vi "log analysis_gps.vi"() -> ()   [LabVIEW 2018] (continued)
471d,15824;INS_ALIGNMENT_COMPLETE,INS_RTKFIXED,37.37103636428,126.72354662832,8.3755,22.3000,0.1350,-0.2615,-0.0053,-0.069883534,-0.948015743,292.302597203,0.4446,0.2951,0.5590,0.1140,0.0925,0.0776,0.0978,0.1028,4.9465,0f000001,0*59130eb8\n\t", "INSPVAXA,USB3,0,51.0,FINESTEERING,2107,283021.700,02000000,471d,15824;INS_ALIGNMENT_COMPLETE,INS_RTKFIXED,37.37105488806,126.72349758761,8.3107,22.3000,0.1124,-0.2877,-0.0191,-0.603845157,-1.428014368,288.935954178,0.4473,0.2957,0.5615,0.1144,0.0929,0.0777,0.0976,0.1028,4.9397,0f000001,0*95301355\n\t", "INSPVAXA,USB3,0,49.5,FINESTEERING,2107,283026.200,02000000,471d,15824;INS_ALIGNMENT_COMPLETE,INS_RTKFIXED,37.37105960737,126.72348434447,8.2980,22.3000,0.1329,-0.2636,-0.0189,0.063004840,-0.340709655,286.479818282,0.4478,0.2967,0.5618,0.1144,0.0930,0.0777,0.0976,0.1028,4.9376,0f000001,0*1276055f\n\t", "INSPVAXA,USB3,0,49.5,FINESTEERING,2107,283026.700,02000000,471d,15824;INS_ALIGNMENT_COMPLETE,INS_RTKFIXED,37.37106011573,126.72348287105,8.2978,22.3000,0.1361,-0.2641,-0.0054,0.117267102,-0.429574615,286.158968157,0.4478,0.2967,0.5618,0.1144,0.0930,0.0777,0.0976,0.1028,4.9376,0f000001,0*5e7b6e4c\n\t", "INSPVAXA,USB3,0,51.0,FINESTEERING,2107,283028.700,02000000,471d,15824;INS_ALIGNMENT_COMPLETE,INS_RTKFIXED,37.37106216690,126.72347687588,8.2864,22.3000,0.1309,-0.2689,-0.0192,0.186843092,-0.733613346,285.184747118,0.4481,0.2969,0.5618,0.1144,0.0930,0.0777,0.0976,0.1028,4.9364,0f000001,0*7469a4e3\n\t", "INSPVAXA,USB3,0,50.5,FINESTEERING,2107,283031.700,02000000,471d,15824;INS_ALIGNMENT_COMPLETE,INS_RTKFIXED,37.37106478537,126.72346780785,8.2718,22.3000,0.1039,-0.2615,-0.0058,0.432632982,-0.697195774,283.403693231,0.4679,0.3078,0.5901,0.1164,0.0946,0.0783,0.0984,0.1034,4.9333,0f000001,0*22ba6c5b\n\t", "INSPVAXA,USB3,0,52.5,FINESTEERING,2107,283032.700,02000000,471d,15824;INS_ALIGNMENT_COMPLETE,INS_RTKFIXED,37.37106557652,126.72346477114,8.2666,22.3000,0.1036,-0.2653,-0.0227,0.510573664,-0.506867752,282.989814532,0.4595,0.3023,0.5832,0.1161,0.0945,0.0778,0.0983,0.1032,4.9326,0f000001,0*f19d58ff\n\t", "INSPVAXA,USB3,0,49.5,FINESTEERING,2107,283033.200,02000000,471d,15824;INS_ALIGNMENT_COMPLETE,INS_RTKFIXED,37.37106596612,126.72346326783,8.2630,22.3000,0.1080,-0.2670,-0.0291,0.451082003,-0.356947315,282.881862782,0.4543,0.2994,0.5774,0.1160,0.0946,0.0775,0.0983,0.1032,4.9319,0f000001,0*26a02b0e\n\t", "INSPVAXA,USB3,0,49.5,FINESTEERING,2107,283033.700,02000000,471d,15824;INS_ALIGNMENT_COMPLETE,INS_RTKFIXED,37.37106635735,126.72346178545,8.2608,22.3000,0.1136,-0.2627,-0.0166,0.359711972,-0.310104269,282.738479610,0.4543,0.2994,0.5774,0.1160,0.0946,0.0775,0.0983,0.1032,4.9319,0f000001,0*88f043a8\n\t", "INSPVAXA,USB3,0,50.0,FINESTEERING,2107,283034.200,02000000,471d,15824;INS_ALIGNMENT_COMPLETE,INS_RTKFIXED,37.37106676961,126.72346024394,8.2592,22.3000,0.1183,-0.2649,-0.0209,0.421889182,-0.508488076,282.654292643,0.4522,0.2981,0.5733,0.1161,0.0947,0.0774,0.0982,0.1031,4.9317,0f000001,0*726c30e6\n\t", "INSPVAXA,USB3,0,50.0,FINESTEERING,2107,283034.700,02000000,471d,15824;INS_ALIGNMENT_COMPLETE,INS_RTKFIXED,37.37106718417,126.72345866239,8.2575,22.3000,0.1236,-0.2716,-0.0253,0.328679874,-0.657327214,282.636912326,0.4522,0.2981,0.5733,0.1161,0.0947,0.0774,0.0982,0.1031,4.9317,0f000001,0*dafccd04\n\t", "INSPVAXA,USB3,0,51.5,FINESTEERING,2107,283035.700,02000000,471d,15824;INS_ALIGNMENT_COMPLETE,INS_RTKFIXED,37.37106801887,126.72345563034,8.2572,22.3000,0.1130,-0.2756,-0.0204,0.415680763,-0.663146302,282.634386607,0.4503,0.2974,0.5697,0.1160,0.0945,0.0774,0.0981,0.1030,4.9320,0f000001,0*eab13697\n\t", "INSPVAXA,USB3,0,40.5,FINESTEERING,2107,283036.200,02000000,471d,15824;INS_ALIGNMENT_COMPLETE,INS_RTKFIXED,37.37106843656,126.72345404474,8.2574,22.3000,0.1206,-0.2843,-0.0254,0.323424961,-0.903914329,282.663197732,0.4498,0.2973,0.5674,0.1161,0.0943,0.0774,0.0979,0.1030,4.9328,0f000001,0*9733e7d0\n\t", "INSPVAXA,USB3,0,40.5,FINESTEERING,2107,283036.700,02000000,471d,15824;INS_ALIGNMENT_COMPLETE,INS_RTKFIXED,37.37106883526,126.72345250109,8.2575,22.3000,0.1230,-0.2819,-0.0264,0.242869357,-1.036611365,282.652291179,0.4498,0.2973,0.5674,0.1161,0.0943,0.0774,0.0979,0.1030,4.9328,0f000001,0*470d739a\n\t", "INSPVAXA,USB3,0,48.5,FINESTEERING,2107,283037.200,02000000,471d,15824;INS_ALIGNMENT_COMPLETE,INS_RTKFIXED,37.37106923446,126.72345098005,8.2563,22.3000,0.1194,-0.2683,-0.0234,0.058649364,-1.081028775,282.621575869,0.4494,0.2971,0.5657,0.1160,0.0940,0.0775,0.0978,0.1029,4.9342,0f000001,0*f5724e44\n\t", "INSPVAXA,USB3,0,48.5,FINESTEERING,2107,283037.700,02000000,471d,15824;INS_ALIGNMENT_COMPLETE,INS_RTKFIXED,37.37106966075,126.72344944048,8.2560,22.3000,0.1291,-0.2596,-0.0199,0.104783484,-1.127316645,282.608621596,0.4494,0.2971,0.5657,0.1160,0.0940,0.0775,0.0978,0.1029,4.9342,0f000001,0*8aba2554\n\t", "INSPVAXA,USB3,0,50.0,FINESTEERING,2107,283039.200,02000000,471d,15824;INS_ALIGNMENT_COMPLETE,INS_RTKFIXED,37.37107093141,126.72344485682,8.2573,22.3000,0.1183,-0.2711,-0.0111,0.295639650,-1.102682519,282.550490605,0.4487,0.2965,0.5633,0.1155,0.0932,0.0777,0.0976,0.1027,4.9372,0f000001,0*f4702847\n\t", "INSPVAXA,USB3,0,50.0,FINESTEERING,2107,283039.700,02000000,471d,15824;INS_ALIGNMENT_COMPLETE,INS_RTKFIXED,37.37107133986,126.72344327017,8.2583,22.3000,0.1271,-0.2797,-0.0164,0.252258898,-1.289319637,282.440116082,0.4487,0.2965,0.5633,0.1155,0.0932,0.0777,0.0976,0.1027,4.9372,0f000001,0*06a83079\n\t", "INSPVAXA,USB3,0,50.0,FINESTEERING,2107,283040.200,02000000,471d,15824;INS_ALIGNMENT_COMPLETE,INS_RTKFIXED,37.37107175331,126.72344170516,8.2593,22.3000,0.1172,-0.2595,-0.0203,0.374259867,-1.387302734,282.178298853,0.4482,0.2962,0.5625,0.1153,0.0929,0.0777,0.0976,0.1026,4.9387,0f000001,0*b656771f\n\t", "INSPVAXA,USB3,0,50.0,FINESTEERING,2107,283040.700,02000000,471d,15824;INS_ALIGNMENT_COMPLETE,INS_RTKFIXED,37.37107213898,126.72344017293,8.2600,22.3000,0.1126,-0.2759,-0.0195,0.475030842,-1.266134141,281.998723158,0.4482,0.2962,0.5625,0.1153,0.0929,0.0777,0.0976,0.1026,4.9387,0f000001,0*1f5b23a7\n\t", "INSPVAXA,USB3,0,45.0,FINESTEERING,2107,283041.200,02000000,471d,15824;INS_ALIGNMENT_COMPLETE,INS_RTKFIXED,37.37107252297,126.72343860548,8.2602,22.3000,0.1112,-0.2748,-0.0176,0.520519283,-1.356863437,281.705665102,0.4477,0.2959,0.5620,0.1149,0.0927,0.0778,0.0976,0.1026,4.9400,0f000001,0*79559378\n\t", "INSPVAXA,USB3,0,45.0,FINESTEERING,2107,283041.700,02000000,471d,15824;INS_ALIGNMENT_COMPLETE,INS_RTKFIXED,37.37107290097,126.72343701394,8.2600,22.3000,0.1062,-0.2671,-0.0203,0.682698215,-1.388086535,281.490437420,0.4477,0.2959,0.5620,0.1149,0.0927,0.0778,0.0976,0.1026,4.9400,0f000001,0*78dbf0af\n\t", "INSPVAXA,USB3,0,45.5,FINESTEERING,2107,283042.200,02000000,471d,15824;INS_ALIGNMENT_COMPLETE,INS_RTKFIXED,37.37107326636,126.72343547606,8.2588,22.3000,0.1093,-0.2758,-0.0183,0.747095346,-1.168799839,281.251721154,0.4473,0.2957,0.5618,0.1147,0.0926,0.0778,0.0976,0.1026,4.9413,0f000001,0*2a17f75d\n\t", "INSPVAXA,USB3,0,45.5,FINESTEERING,2107,283042.700,02000000,471d,15824;INS_ALIGNMENT_COMPLETE,INS_RTKFIXED,37.37107361520,126.72343393571,8.2583,22.3000,0.0948,-0.2791,-0.0077,0.665887497,-1.134840592,281.023360507,0.4473,0.2957,0.5618,0.1147,0.0926,0.0778,0.0976,0.1026,4.9413,0f000001,0*de2961a5\n\t", "INSPVAXA,USB3,0,45.5,FINESTEERING,2107,283043.200,02000000,471d,15824;INS_ALIGNMENT_COMPLETE,INS_RTKFIXED,37.37107395395,126.72343236915,8.2577,22.3000,0.0931,-0.2659,-0.0049,0.487857559,-1.159051865,280.826329079,0.4472,0.2955,0.5619,0.1145,0.0925,0.0779,0.0977,0.1026,4.9425,0f000001,0*06efa692\n\t", "INSPVAXA,USB3,0,45.5,FINESTEERING,2107,283043.700,02000000,471d,15824;INS_ALIGNMENT_COMPLETE,INS_RTKFIXED,37.37107428662,126.72343081441,8.2573,22.3000,0.0965,-0.2862,-0.0130,0.491699784,-1.201692637,280.563355107,0.4472,0.2955,0.5619,0.1145,0.0925,0.0779,0.0977,0.1026,4.9425,0f000001,0*ec772638\n\t", "INSPVAXA,USB3,0,49.5,FINESTEERING,2107,283044.200,02000000,471d,15824;INS_ALIGNMENT_COMPLETE,INS_RTKFIXED,37.37107460279,126.72342927244,8.2555,22.3000,0.0952,-0.2841,-0.0084,0.223988399,-1.263049890,280.433215030,0.4470,0.2954,0.5621,0.1143,0.0926,0.0779,0.0977,0.1026,4.9439,0f000001,0*7d3e34bc\n\t", "INSPVAXA,USB3,0,49.5,FINESTEERING,2107,283044.700,02000000,471d,15824;INS_ALIGNMENT_COMPLETE,INS_RTKFIXED,37.37107493652,126.72342768887,8.2530,22.3000,0.0917,-0.2710,-0.0218,0.103359627,-1.313771088,280.424386340,0.4470,0.2954,0.5621,0.1143,0.0926,0.0779,0.0977,0.1026,4.9439,0f000001,0*15507eb4\n\t", "INSPVAXA,USB3,0,50.5,FINESTEERING,2107,283045.200,02000000,471d,15824;INS_ALIGNMENT_COMPLETE,INS_RTKFIXED,37.37107528342,126.72342611252,8.2498,22.3000,0.0937,-0.2667,-0.0213,0.106140982,-1.381356715,280.387415743,0.4469,0.2952,0.5622,0.1142,0.0926,0.0779,0.0977,0.1027,4.9453,0f000001,0*b33463af\n\t", "INSPVAXA,USB3,0,50.5,FINESTEERING,2107,283045.700,02000000,471d,15824;INS_ALIGNMENT_COMPLETE,INS_RTKFIXED,37.37107563193,126.72342458286,8.2474,22.3000,0.0924,-0.2735,-0.0177,0.170304952,-1.470111743,280.394073740,0.4469,0.2952,0.5622,0.1142,0.0926,0.0779,0.0977,0.1027,4.9453,0f000001,0*1961b7fd\n\t", "INSPVAXA,USB3,0,50.5,FINESTEERING,2107,283046.200,02000000,471d,15824;INS_ALIGNMENT_COMPLETE,INS_RTKFIXED,37.37107597691,126.72342305519,8.2441,22.3000,0.1009,-0.2727,-0.0163,0.064516230,-1.445309822,280.441255220,0.4468,0.2952,0.5622,0.1142,0.0926,0.0779,0.0977,0.1027,4.9463,0f000001,0*2fb8f12d\n\t", "INSPVAXA,USB3,0,50.5,FINESTEERING,2107,283046.700,02000000,471d,15824;INS_ALIGNMENT_COMPLETE,INS_RTKFIXED,37.37107633807,126.72342148609,8.2393,22.3000,0.0964,-0.2701,-0.0237,0.142828427,-1.613985055,280.469492916,0.4468,0.2952,0.5622,0.1142,0.0926,0.0779,0.0977,0.1027,4.9463,0f000001,0*98edc3e5\n\t", "INSPVAXA,USB3,0,51.0,FINESTEERING,2107,283047.200,02000000,471d,15824;INS_ALIGNMENT_COMPLETE,INS_RTKFIXED,37.37107668709,126.72341995437,8.2353,22.3000,0.0927,-0.2633,-0.0258,0.010167454,-1.546701377,280.494856873,0.4468,0.2952,0.5623,0.1142,0.0927,0.0779,0.0977,0.1028,4.9471,0f000001,0*6fb0fd0d\n\t", "INSPVAXA,USB3,0,51.0,FINESTEERING,2107,283047.700,02000000,471d,15824;INS_ALIGNMENT_COMPLETE,INS_RTKFIXED,37.37107702961,126.72341848936,8.2340,22.3000,0.0963,-0.2679,-0.0257,0.001855502,-1.278269974,280.498870950,0.4468,0.2952,0.5623,0.1142,0.0927,0.0779,0.0977,0.1028,4.9471,0f000001,0*57b2ac91\n\t", "INSPVAXA,USB3,0,51.0,FINESTEERING,2107,283048.200,02000000,471d,15824;INS_ALIGNMENT_COMPLETE,INS_RTKFIXED,37.37107738369,126.72341697976,8.2314,22.3000,0.0870,-0.2415,-0.0190,0.047758290,-1.244931408,280.498951472,0.4468,0.2952,0.5625,0.1142,0.0926,0.0779,0.0977,0.1028,4.9478,0f000001,0*d01a0722\n\t", "INSPVAXA,USB3,0,51.0,FINESTEERING,2107,283048.700,02000000,471d,15824;INS_ALIGNMENT_COMPLETE,INS_RTKFIXED,37.37107774021,126.72341542793,8.2273,22.3000,0.0934,-0.2612,-0.0233,0.100861345,-1.232017596,280.548708433,0.4468,0.2952,0.5625,0.1142,0.0926,0.0779,0.0977,0.1028,4.9478,0f000001,0*f829d1eb\n\t", "INSPVAXA,USB3,0,51.5,FINESTEERING,2107,283049.200,02000000,471d,15824;INS_ALIGNMENT_COMPLETE,INS_RTKFIXED,37.37107809495,126.72341393568,8.2249,22.3000,0.0985,-0.2703,-0.0295,0.221283092,-1.050797782,280.593013812,0.4472,0.2952,0.5628,0.1144,0.0926,0.0779,0.0977,0.1029,4.9484,0f000001,0*0fbf0092\n\t", "INSPVAXA,USB3,0,51.5,FINESTEERING,2107,283049.700,02000000,471d,15824;INS_ALIGNMENT_COMPLETE,INS_RTKFIXED,37.37107844035,126.72341241620,8.2243,22.3000,0.0876,-0.2464,-0.0197,0.278290436,-1.204720693,280.644287855,0.4472,0.2952,0.5628,0.1144,0.0926,0.0779,0.0977,0.1029,4.9484,0f000001,0*062abefc\n\t", "DUALANTENNAHEADINGA,USB3,0,46.0,FINESTEERING,2107,283050.200,02000000,d426,15824;INSUFFICIENT_OBS,NONE,-1.000000000,0.000000000,0.000000000,0.0,0.000000000,0.000000000,\"631T\",16,2,2,2,04,00,20,00*50cdafe2\n\t", "INSPVAXA,USB3,0,46.0,FINESTEERING,2107,283050.700,02000000,471d,15824;INS_ALIGNMENT_COMPLETE,INS_RTKFIXED,37.37107913318,126.72340926618,8.2224,22.3000,0.0989,-0.2842,-0.0266,-0.029207356,-1.258376136,280.779017967,0.4478,0.2954,0.5630,0.1143,0.0926,0.0779,0.0977,0.1029,4.9492,0f000001,0*5132ab61\n\t", "DUALANTENNAHEADINGA,USB3,0,49.5,FINESTEERING,2107,283051.200,02000000,d426,15824;INSUFFICIENT_OBS,NONE,-1.000000000,0.000000000,0.000000000,0.0,0.000000000,0.000000000,\"631T\",13,2,2,2,04,00,20,00*248e5ed2\n\t", "DUALANTENNAHEADINGA,USB3,0,49.5,FINESTEERING,2107,283051.700,02000000,d426,15824;INSUFFICIENT_OBS,NONE,-1.000000000,0.000000000,0.000000000,0.0,0.000000000,0.000000000,\"631T\",14,2,2,2,04,00,20,00*b9a3c4c0\n\t", "INSPVAXA,USB3,0,50.5,FINESTEERING,2107,283052.200,02000000,471d,15824;INS_ALIGNMENT_COMPLETE,INS_RTKFIXED,37.37108016490,126.72340456105,8.2187,22.3000,0.0964,-0.2582,-0.0125,0.437479141,-1.522113424,279.604758230,0.4484,0.2957,0.5640,0.1144,0.0927,0.0779,0.0976,0.1029,4.9509,0f000001,0*77064c2d\n\t", "INSPVAXA,USB3,0,50.5,FINESTEERING,2107,283052.700,02000000,471d,15824;INS_ALIGNMENT_COMPLETE,INS_RTKFIXED,37.37108046861,126.72340298306,8.2170,22.3000,0.0891,-0.2658,-0.0140,0.468373429,-1.552166741,279.130645467,0.4484,0.2957,0.5640,0.1144,0.0927,0.0779,0.0976,0.1029,4.9509,0f000001,0*1c6e477e\n\t", "INSPVAXA,USB3,0,48.5,FINESTEERING,2107,283053.200,02000000,471d,15824;INS_ALIGNMENT_COMPLETE,INS_RTKFIXED,37.37108075231,126.72340140427,8.2151,22.3000,0.0764,-0.2907,-0.0105,0.358370725,-1.600173784,278.606485761,0.4480,0.2956,0.5639,0.1143,0.0926,0.0779,0.0976,0.1029,4.9518,0f000001,0*3a7eab6c\n\t", "INSPVAXA,USB3,0,48.5,FINESTEERING,2107,283053.700,02000000,471d,15824;INS_ALIGNMENT_COMPLETE,INS_RTKFIXED,37.37108102802,126.72339980538,8.2112,22.3000,0.0729,-0.2744,-0.0174,0.330552076,-1.494765101,278.139995916,0.4480,0.2956,0.5639,0.1143,0.0926,0.0779,0.0976,0.1029,4.9518,0f000001,0*6b892211\n\t", "DUALANTENNAHEADINGA,USB3,0,45.5,FINESTEERING,2107,283054.200,02000000,d426,15824;INSUFFICIENT_OBS,NONE,-1.000000000,0.000000000,0.000000000,0.0,0.000000000,0.000000000,\"631T\",19,2,2,2,04,00,20,00*86f4b129\n\t", "INSPVAXA,USB3,0,45.5,FINESTEERING,2107,283054.700,02000000,471d,15824;INS_ALIGNMENT_COMPLETE,INS_RTKFIXED,37.37108154829,126.72339665209,8.2035,22.3000,0.0578,-0.2607,-0.0176,0.280593250,-1.428439620,277.446082188,0.4484,0.2957,0.5646,0.1144,0.0926,0.0779,0.0976,0.1029,4.9527,0f000001,0*8d0f64c8\n\t", "INSPVAXA,USB3,0,46.0,FINESTEERING,2107,283055.200,02000000,471d,15824;INS_ALIGNMENT_COMPLETE,INS_RTKFIXED,37.37108179458,126.72339508506,8.2008,22.3000,0.0590,-0.2687,-0.0093,0.251526173,-1.446507840,277.289322874,0.4481,0.2956,0.5644,0.1143,0.0926,0.0779,0.0976,0.1029,4.9538,0f000001,0*05040f15\n\t", "INSPVAXA,USB3,0,46.0,FINESTEERING,2107,283055.700,02000000,471d,15824;INS_ALIGNMENT_COMPLETE,INS_RTKFIXED,37.37108204101,126.72339350294,8.1980,22.3000,0.0573,-0.2710,-0.0141,0.338881932,-1.408720439,277.315135363,0.4481,0.2956,0.5644,0.1143,0.0926,0.0779,0.0976,0.1029,4.9538,0f000001,0*6debbe04\n\t", "INSPVAXA,USB3,0,52.0,FINESTEERING,2107,283056.200,02000000,471d,15824;INS_ALIGNMENT_COMPLETE,INS_RTKFIXED,37.37108228588,126.72339196103,8.1952,22.3000,0.0487,-0.2508,-0.0076,0.405017158,-1.170976426,277.337977168,0.4477,0.2956,0.5639,0.1144,0.0926,0.0778,0.0976,0.1028,4.9548,0f000001,0*8b541580\n\t", "DUALANTENNAHEADINGA,USB3,0,52.0,FINESTEERING,2107,283056.700,02000000,d426,15824;INSUFFICIENT_OBS,NONE,-1.000000000,0.000000000,0.000000000,0.0,0.000000000,0.000000000,\"631T\",13,2,2,2,04,00,20,00*95485060\n\t", "DUALANTENNAHEADINGA,USB3,0,50.0,FINESTEERING,2107,283057.200,02000000,d426,15824;INSUFFICIENT_OBS,NONE,-1.000000000,0.000000000,0.000000000,0.0,0.000000000,0.000000000,\"631T\",13,2,2,2,04,00,20,00*e70ae8a8\n\t", "DUALANTENNAHEADINGA,USB3,0,50.0,FINESTEERING,2107,283057.700,02000000,d426,15824;INSUFFICIENT_OBS,NONE,-1.000000000,0.000000000,0.000000000,0.0,0.000000000,0.000000000,\"631T\",13,2,2,2,04,00,20,00*3019f9f1\n\t", "INSPVAXA,USB3,0,52.0,FINESTEERING,2107,283058.200,02000000,471d,15824;INS_ALIGNMENT_COMPLETE,INS_RTKFIXED,37.37108315467,126.72338641713,8.1848,22.3000,0.0560,-0.2718,-0.0107,0.129590736,-0.819774204,277.698102716,0.4474,0.2955,0.5631,0.1155,0.0927,0.0778,0.0975,0.1028,4.9554,0f000001,0*a6d9a945\n\t", "INSPVAXA,USB3,0,52.0,FINESTEERING,2107,283058.700,02000000,471d,15824;INS_ALIGNMENT_COMPLETE,INS_RTKFIXED,37.37108344441,126.72338455262,8.1832,22.3000,0.0621,-0.2653,-0.0184,0.032268015,-0.987434909,277.857905932,0.4474,0.2955,0.5631,0.1155,0.0927,0.0778,0.0975,0.1028,4.9554,0f000001,0*0fff6d0e\n\t", "INSPVAXA,USB3,0,51.0,FINESTEERING,2107,283059.200,02000000,471d,15824;INS_ALIGNMENT_COMPLETE,INS_RTKFIXED,37.37108373104,126.72338298116,8.1814,22.3000,0.0640,-0.2840,-0.0248,0.084962299,-0.861930897,278.528163453,0.4480,0.2954,0.5625,0.1142,0.0926,0.0777,0.0975,0.1027,4.9533,0f000001,0*55180826\n\t", "INSPVAXA,USB3,0,51.0,FINESTEERING,2107,283059.700,02000000,471d,15824;INS_ALIGNMENT_COMPLETE,INS_RTKFIXED,37.37108405973,126.72338145683,8.1789,22.3000,0.0766,-0.2838,-0.0077,0.302314246,-0.745003967,279.694826311,0.4480,0.2954,0.5625,0.1142,0.0926,0.0777,0.0975,0.1027,4.9533,0f000001,0*c3a85521\n\t", "DUALANTENNAHEADINGA,USB3,0,49.5,FINESTEERING,2107,283060.200,02000000,d426,15824;INSUFFICIENT_OBS,NONE,-1.000000000,0.000000000,0.000000000,0.0,0.000000000,0.000000000,\"631T\",14,2,2,2,04,00,20,00*d9be019d\n\t", "INSPVAXA,USB3,0,49.5,FINESTEERING,2107,283060.700,02000000,471d,15824;INS_ALIGNMENT_COMPLETE,INS_RTKFIXED,37.37108477080,126.72337829109,8.1755,22.3000,0.0829,-0.2746,-0.0191,-0.114275154,-0.865621982,282.712324181,0.4478,0.2952,0.5620,0.1144,0.0926,0.0777,0.0975,0.1027,4.9522,0f000001,0*f5ce6e6a\n\t", "DUALANTENNAHEADINGA,USB3,0,49.0,FINESTEERING,2107,283061.200,02008000,d426,15824;SOL_COMPUTED,L1_FLOAT,-1.000000000,252.567794800,53.338584900,0.0,294.937744141,135.460769653,\"631T\",15,6,6,6,04,00,20,23*fbe42f58\n\t", "DUALANTENNAHEADINGA,USB3,0,49.0,FINESTEERING,2107,283061.700,02008000,d426,15824;INSUFFICIENT_OBS,NONE,-1.000000000,0.000000000,0.000000000,0.0,0.000000000,0.000000000,\"631T\",13,2,2,2,04,00,20,00*6aa2fd3b\n\t", "DUALANTENNAHEADINGA,USB3,0,45.5,FINESTEERING,2107,283062.200,02008000,d426,15824;INSUFFICIENT_OBS,NONE,-1.000000000,0.000000000,0.000000000,0.0,0.000000000,0.000000000,\"631T\",13,2,2,2,04,00,20,00*8005e2b6\n\t", "DUALANTENNAHEADINGA,USB3,0,45.5,FINESTEERING,2107,283062.700,02008000,d426,15824;INSUFFICIENT_OBS,NONE,-1.000000000,0.000000000,0.000000000,0.0,0.000000000,0.000000000,\"631T\",13,2,2,2,04,00,20,00*5716f3ef\n\t", "DUALANTENNAHEADINGA,USB3,0,46.0,FINESTEERING,2107,283063.200,02008000,d426,15824;INSUFFICIENT_OBS,NONE,-1.000000000,0.000000000,0.000000000,0.0,0.000000000,0.000000000,\"631T\",12,2,2,2,04,00,20,00*c388fb17\n\t", "INSPVAXA,USB3,0,46.0,FINESTEERING,2107,283063.700,02008000,471d,15824;INS_ALIGNMENT_COMPLETE,INS_RTKFIXED,37.37108763910,126.72336915850,8.1772,22.3000,0.0613,-0.1484,-0.0057,-0.315544156,-0.705788351,288.188502375,0.4460,0.2952,0.5608,0.1140,0.0926,0.0776,0.0975,0.1026,4.9515,0f000001,0*11521a0a\n\t", "DUALANTENNAHEADINGA,USB3,0,49.5,FINESTEERING,2107,283064.200,02008000,d426,15824;INSUFFICIENT_OBS,NONE,-1.000000000,0.000000000,0.000000000,0.0,0.000000000,0.000000000,\"631T\",14,2,2,2,04,00,20,00*a33c9019\n\t", "DUALANTENNAHEADINGA,USB3,0,49.5,FINESTEERING,2107,283064.700,02008000,d426,15824;INSUFFICIENT_OBS,NONE,-1.000000000,0.000000000,0.000000000,0.0,0.000000000,0.000000000,\"631T\",13,2,2,2,04,00,20,00*3e110a0b\n\t", "DUALANTENNAHEADINGA,USB3,0,50.0,FINESTEERING,2107,283065.200,02008000,d426,15824;INSUFFICIENT_OBS,NONE,-1.000000000,0.000000000,0.000000000,0.0,0.000000000,0.000000000,\"631T\",13,2,2,2,04,00,20,00*f0ffb566\n\t", "DUALANTENNAHEADINGA,USB3,0,50.0,FINESTEERING,2107,283065.700,02008000,d426,15824;INSUFFICIENT_OBS,NONE,-1.000000000,0.000000000,0.000000000,0.0,0.000000000,0.000000000,\"631T\",14,2,2,2,04,00,20,00*6dd22f74\n\t", "DUALANTENNAHEADINGA,USB3,0,47.5,FINESTEERING,2107,283066.200,02000000,d426,15824;INSUFFICIENT_OBS,NONE,-1.000000000,0.000000000,0.000000000,0.0,0.000000000,0.000000000,\"631T\",15,2,2,2,04,00,20,00*afd2d569\n\t", "INSPVAXA,USB3,0,47.5,FINESTEERING,2107,283066.700,02000000,471d,15824;INS_ALIGNMENT_COMPLETE,INS_RTKFIXED,37.37108811035,126.72336925303,8.1815,22.3000,0.0201,0.0148,-0.0079,-0.417962669,-0.573305874,287.968672901,0.4491,0.2953,0.5602,0.1160,0.0930,0.0776,0.0974,0.1026,4.9384,0f000001,0*010a2d8b\n\t", "INSPVAXA,USB3,0,49.5,FINESTEERING,2107,283067.200,02000000,471d,15824;INS_ALIGNMENT_COMPLETE,INS_RTKFIXED,37.37108813168,126.72336927578,8.1822,22.3000,0.0181,0.0163,-0.0073,-0.419452547,-0.574416189,287.977918899,0.4495,0.2954,0.5600,0.1153,0.0929,0.0776,0.0974,0.1026,4.9275,0f000001,0*549c769b\n\t", "DUALANTENNAHEADINGA,USB3,0,49.5,FINESTEERING,2107,283067.700,02000000,d426,15824;INSUFFICIENT_OBS,NONE,-1.000000000,0.000000000,0.000000000,0.0,0.000000000,0.000000000,\"631T\",12,2,2,2,04,00,20,00*49080399\n\t", "DUALANTENNAHEADINGA,USB3,0,52.0,FINESTEERING,2107,283068.200,02000000,d426,15824;INSUFFICIENT_OBS,NONE,-1.000000000,0.000000000,0.000000000,0.0,0.000000000,0.000000000,\"631T\",10,2,2,2,04,00,20,00*54582190\n\t", "DUALANTENNAHEADINGA,USB3,0,52.0,FINESTEERING,2107,283068.700,02000000,d426,15824;INSUFFICIENT_OBS,NONE,-1.000000000,0.000000000,0.000000000,0.0,0.000000000,0.000000000,\"631T\",10,2,2,2,04,00,20,00*834b30c9\n\t", "DUALANTENNAHEADINGA,USB3,0,51.0,FINESTEERING,2107,283069.200,02000000,d426,15824;INSUFFICIENT_OBS,NONE,-1.000000000,0.000000000,0.000000000,0.0,0.000000000,0.000000000,\"631T\",10,2,2,2,04,00,20,00*954d5ea5\n\t", "DUALANTENNAHEADINGA,USB3,0,51.0,FINESTEERING,2107,283069.700,02000000,d426,15824;INSUFFICIENT_OBS,NONE,-1.000000000,0.000000000,0.000000000,0.0,0.000000000,0.000000000,\"631T\",10,2,2,2,04,00,20,00*425e4ffc\n\t", "DUALANTENNAHEADINGA,USB3,0,52.5,FINESTEERING,2107,283070.200,02000000,d426,15824;INSUFFICIENT_OBS,NONE,-1.000000000,0.000000000,0.000000000,0.0,0.000000000,0.000000000,\"631T\",10,2,2,2,04,00,20,00*26625f62\n\t", "DUALANTENNAHEADINGA,USB3,0,52.5,FINESTEERING,2107,283070.700,02000000,d426,15824;INSUFFICIENT_OBS,NONE,-1.000000000,0.000000000,0.000000000,0.0,0.000000000,0.000000000,\"631T\",13,2,2,2,04,00,20,00*5227c892\n\t", "DUALANTENNAHEADINGA,USB3,0,54.5,FINESTEERING,2107,283071.200,02000000,d426,15824;INSUFFICIENT_OBS,NONE,-1.000000000,0.000000000,0.000000000,0.0,0.000000000,0.000000000,\"631T\",13,2,2,2,04,00,20,00*6a072c8b\n\t", "DUALANTENNAHEADINGA,USB3,0,49.5,FINESTEERING,2107,283072.200,02000000,d426,15824;INSUFFICIENT_OBS,NONE,-1.000000000,0.000000000,0.000000000,0.0,0.000000000,0.000000000,\"631T\",11,2,2,2,04,00,20,00*c3e637e1\n\t", "DUALANTENNAHEADINGA,USB3,0,49.5,FINESTEERING,2107,283072.700,02000000,d426,15824;INSUFFICIENT_OBS,NONE,-1.000000000,0.000000000,0.000000000,0.0,0.000000000,0.000000000,\"631T\",13,2,2,2,04,00,20,00*60412049\n\t", "DUALANTENNAHEADINGA,USB3,0,45.5,FINESTEERING,2107,283073.200,02000000,d426,15824;INSUFFICIENT_OBS,NONE,-1.000000000,0.000000000,0.000000000,0.0,0.000000000,0.000000000,\"631T\",13,2,2,2,04,00,20,00*042cd0ba\n\t", "DUALANTENNAHEADINGA,USB3,0,45.5,FINESTEERING,2107,283073.700,02000000,d426,15824;INSUFFICIENT_OBS,NONE,-1.000000000,0.000000000,0.000000000,0.0,0.000000000,0.000000000,\"631T\",14,2,2,2,04,00,20,00*99014aa8\n\t", "DUALANTENNAHEADINGA,USB3,0,50.0,FINESTEERING,2107,283074.200,02000000,d426,15824;INSUFFICIENT_OBS,NONE,-1.000000000,0.000000000,0.000000000,0.0,0.000000000,0.000000000,\"631T\",14,2,2,2,04,00,20,00*3ee80c21\n\t", "DUALANTENNAHEADINGA,USB3,0,50.0,FINESTEERING,2107,283074.700,02000000,d426,15824;INSUFFICIENT_OBS,NONE,-1.000000000,0.000000000,0.000000000,0.0,0.000000000,0.000000000,\"631T\",13,2,2,2,04,00,20,00*a3c59633\n\t", "DUALANTENNAHEADINGA,USB3,0,48.5,FINESTEERING,2107,283075.200,02000000,d426,15824;INSUFFICIENT_OBS,NONE,-1.000000000,0.000000000,0.000000000,0.0,0.000000000,0.000000000,\"631T\",14,2,2,2,04,00,20,00*435174b1\n\t", "DUALANTENNAHEADINGA,USB3,0,48.5,FINESTEERING,2107,283075.700,02000000,d426,15824;INSUFFICIENT_OBS,NONE,-1.000000000,0.000000000,0.000000000,0.0,0.000000000,0.000000000,\"631T\",14,2,2,2,04,00,20,00*944265e8\n\t", "DUALANTENNAHEADINGA,USB3,0,37.5,FINESTEERING,2107,283076.200,02000000,d426,15824;INSUFFICIENT_OBS,NONE,-1.000000000,0.000000000,0.000000000,0.0,0.000000000,0.000000000,\"631T\",12,2,2,2,04,00,20,00*42000f60\n\t", "DUALANTENNAHEADINGA,USB3,0,37.5,FINESTEERING,2107,283076.700,02000000,d426,15824;INSUFFICIENT_OBS,NONE,-1.000000000,0.000000000,0.000000000,0.0,0.000000000,0.000000000,\"631T\",12,2,2,2,04,00,20,00*95131e39\n\t", "DUALANTENNAHEADINGA,USB3,0,41.5,FINESTEERING,2107,283077.200,02000000,d426,15824;INSUFFICIENT_OBS,NONE,-1.000000000,0.000000000,0.000000000,0.0,0.000000000,0.000000000,\"631T\",13,2,2,2,04,00,20,00*225f994e\n\t", "DUALANTENNAHEADINGA,USB3,0,41.5,FINESTEERING,2107,283077.700,02000000,d426,15824;INSUFFICIENT_OBS,NONE,-1.000000000,0.000000000,0.000000000,0.0,0.000000000,0.000000000,\"631T\",14,2,2,2,04,00,20,00*bf72035c\n\t", "DUALANTENNAHEADINGA,USB3,0,47.5,FINESTEERING,2107,283078.700,02000000,d426,15824;INSUFFICIENT_OBS,NONE,-1.000000000,0.000000000,0.000000000,0.0,0.000000000,0.000000000,\"631T\",14,2,2,2,04,00,20,00*3fc2c0c1\n\t", "INSPVAXA,USB3,0,47.0,FINESTEERING,2107,283079.250,02008000,471d,15824;INS_ALIGNMENT_COMPLETE,INS_RTKFIXED,37.37108788068,126.72336895793,8.2189,22.3000,0.0088,0.0013,-0.0012,-0.401485866,-0.591652619,287.973728649,0.2375,0.1652,0.3301,0.0344,0.0343,0.0312,0.0796,0.0806,4.8842,0f000005,0*b7c6e88e\n\t", "DUALANTENNAHEADINGA,USB3,0,48.5,FINESTEERING,2107,283080.200,02008000,d426,15824;INSUFFICIENT_OBS,NONE,-1.000000000,0.000000000,0.000000000,0.0,0.000000000,0.000000000,\"631T\",14,2,2,2,04,00,20,00*53647ec7\n\t", "DUALANTENNAHEADINGA,USB3,0,49.5,FINESTEERING,2107,283081.200,02008000,d426,15824;INSUFFICIENT_OBS,NONE,-1.000000000,0.000000000,0.000000000,0.0,0.000000000,0.000000000,\"631T\",13,2,2,2,04,00,20,00*10c627f1\n\t", "DUALANTENNAHEADINGA,USB3,0,49.5,FINESTEERING,2107,283081.700,02008000,d426,15824;INSUFFICIENT_OBS,NONE,-1.000000000,0.000000000,0.000000000,0.0,0.000000000,0.000000000,\"631T\",13,2,2,2,04,00,20,00*c7d536a8\n\t", "INSPVAXA,USB3,0,48.0,FINESTEERING,2107,283082.250,02008000,471d,15824;INS_ALIGNMENT_COMPLETE,INS_RTKFIXED,37.37108790543,126.72336897434,8.2212,22.3000,0.0087,0.0020,-0.0010,-0.406487889,-0.586741608,287.950772341,0.2277,0.1614,0.3135,0.0344,0.0343,0.0312,0.0796,0.0806,4.8871,0f000005,0*4c1cc0b2\n\t", "DUALANTENNAHEADINGA,USB3,0,48.0,FINESTEERING,2107,283082.700,02008000,d426,15824;INSUFFICIENT_OBS,NONE,-1.000000000,0.000000000,0.000000000,0.0,0.000000000,0.000000000,\"631T\",13,2,2,2,04,00,20,00*40830bab\n\t", "DUALANTENNAHEADINGA,USB3,0,51.0,FINESTEERING,2107,283083.200,02008000,d426,15824;INSUFFICIENT_OBS,NONE,-1.000000000,0.000000000,0.000000000,0.0,0.000000000,0.000000000,\"631T\",13,2,2,2,04,00,20,00*db17520a\n\t", "INSPVAXA,USB3,0,51.0,FINESTEERING,2107,283083.750,02008000,471d,15824;INS_ALIGNMENT_COMPLETE,INS_RTKFIXED,37.37108791341,126.72336897923,8.2220,22.3000,0.0085,0.0022,-0.0015,-0.407747547,-0.586428741,287.947615621,0.2254,0.1606,0.3090,0.0344,0.0343,0.0312,0.0797,0.0806,4.8884,0f000005,0*f8c3e66c\n\t", "DUALANTENNAHEADINGA,USB3,0,45.5,FINESTEERING,2107,283084.200,02008000,d426,15824;INSUFFICIENT_OBS,NONE,-1.000000000,0.000000000,0.000000000,0.0,0.000000000,0.000000000,\"631T\",11,2,2,2,04,00,20,00*bb1dd58f\n\t", "DUALANTENNAHEADINGA,USB3,0,52.0,FINESTEERING,2107,283085.700,02008000,d426,15824;INSUFFICIENT_OBS,NONE,-1.000000000,0.000000000,0.000000000,0.0,0.000000000,0.000000000,\"631T\",13,2,2,2,04,00,20,00*17682428\n\t", "DUALANTENNAHEADINGA,USB3,0,48.5,FINESTEERING,2107,283086.200,02008000,d426,15824;INSUFFICIENT_OBS,NONE,-1.000000000,0.000000000,0.000000000,0.0,0.000000000,0.000000000,\"631T\",11,2,2,2,04,00,20,00*da4fefea\n\t", "INSPVAXA,USB3,0,48.5,FINESTEERING,2107,283086.750,02008000,471d,15824;INS_ALIGNMENT_COMPLETE,INS_RTKFIXED,37.37108790964,126.72336897431,8.2231,22.3000,0.0055,-0.0003,-0.0011,-0.414418876,-0.584788673,287.941437407,0.2201,0.1591,0.2978,0.0344,0.0343,0.0312,0.0796,0.0806,4.8926,0f000005,0*39edc872\n\t", "INSPVAXA,USB3,0,50.0,FINESTEERING,2107,283087.250,02000000,471d,15824;INS_ALIGNMENT_COMPLETE,INS_RTKFIXED,37.37108790633,126.72336897138,8.2235,22.3000,0.0050,-0.0003,-0.0013,-0.412674863,-0.583241565,287.941135781,0.2189,0.1588,0.2948,0.0344,0.0343,0.0312,0.0796,0.0806,4.8941,0f000005,0*d8c4a8b8\n\t", "INSPVAXA,USB3,0,50.0,FINESTEERING,2107,283087.750,02000000,471d,15824;INS_ALIGNMENT_COMPLETE,INS_RTKFIXED,37.37108790910,126.72336896298,8.2239,22.3000,0.0060,-0.0018,-0.0010,-0.411196763,-0.583056579,287.939929568,0.2189,0.1588,0.2948,0.0344,0.0343,0.0312,0.0796,0.0806,4.8941,0f000005,0*cc42fb84\n\t", "INSPVAXA,USB3,0,51.5,FINESTEERING,2107,283088.750,02000000,471d,15824;INS_ALIGNMENT_COMPLETE,INS_RTKFIXED,37.37108791273,126.72336896374,8.2243,22.3000,0.0059,-0.0008,-0.0019,-0.408020685,-0.578100141,287.936827542,0.2178,0.1585,0.2920,0.0344,0.0343,0.0312,0.0796,0.0806,4.8955,0f000005,0*8a62d2d3\n\t", "DUALANTENNAHEADINGA,USB3,0,50.5,FINESTEERING,2107,283089.200,02000000,d426,15824;INSUFFICIENT_OBS,NONE,-1.000000000,0.000000000,0.000000000,0.0,0.000000000,0.000000000,\"631T\",11,2,2,2,04,00,20,00*8b9cc3ca\n\t", "DUALANTENNAHEADINGA,USB3,0,50.5,FINESTEERING,2107,283089.700,02000000,d426,15824;INSUFFICIENT_OBS,NONE,-1.000000000,0.000000000,0.000000000,0.0,0.000000000,0.000000000,\"631T\",12,2,2,2,04,00,20,00*ffd9543a\n\t", "INSPVAXA,USB3,0,48.0,FINESTEERING,2107,283090.250,02000000,471d,15824;INS_ALIGNMENT_COMPLETE,INS_RTKFIXED,37.37108791260,126.72336897396,8.2253,22.3000,0.0056,0.0014,-0.0008,-0.404918336,-0.579813079,287.934409966,0.2159,0.1581,0.2871,0.0344,0.0343,0.0312,0.0796,0.0806,4.8985,0f000005,0*237dfef6\n\t", "INSPVAXA,USB3,0,48.0,FINESTEERING,2107,283090.750,02000000,471d,15824;INS_ALIGNMENT_COMPLETE,INS_RTKFIXED,37.37108791340,126.72336897831,8.2257,22.3000,0.0060,0.0017,-0.0005,-0.406200324,-0.580436127,287.932734672,0.2159,0.1581,0.2871,0.0344,0.0343,0.0312,0.0796,0.0806,4.8985,0f000005,0*2244ce35\n\t", "DUALANTENNAHEADINGA,USB3,0,52.0,FINESTEERING,2107,283091.200,02000000,d426,15824;INSUFFICIENT_OBS,NONE,-1.000000000,0.000000000,0.000000000,0.0,0.000000000,0.000000000,\"631T\",10,2,2,2,04,00,20,00*e6cd9028\n\t", "INSPVAXA,USB3,0,52.0,FINESTEERING,2107,283091.750,02000000,471d,15824;INS_ALIGNMENT_COMPLETE,INS_RTKFIXED,37.37108791121,126.72336898157,8.2259,22.3000,0.0063,0.0022,-0.0001,-0.406191825,-0.576334644,287.931619498,0.2151,0.1580,0.2849,0.0344,0.0343,0.0312,0.0796,0.0806,4.9000,0f000005,0*09e92407\n\t", "DUALANTENNAHEADINGA,USB3,0,46.5,FINESTEERING,2107,283092.200,02008000,d426,15824;INSUFFICIENT_OBS,NONE,-1.000000000,0.000000000,0.000000000,0.0,0.000000000,0.000000000,\"631T\",12,2,2,2,04,00,20,00*fc458629\n\t", "INSPVAXA,USB3,0,46.5,FINESTEERING,2107,283092.750,02008000,471d,15824;INS_ALIGNMENT_COMPLETE,INS_RTKFIXED,37.37108790953,126.72336899162,8.2261,22.3000,0.0061,0.0038,0.0006,-0.405842887,-0.574777504,287.928097277,0.2145,0.1579,0.2830,0.0344,0.0343,0.0312,0.0796,0.0806,4.9014,0f000005,0*3b1b2e95\n\t", "DUALANTENNAHEADINGA,USB3,0,46.5,FINESTEERING,2107,283093.200,02008000,d426,15824;INSUFFICIENT_OBS,NONE,-1.000000000,0.000000000,0.000000000,0.0,0.000000000,0.000000000,\"631T\",12,2,2,2,04,00,20,00*919d82f0\n\t", "INSPVAXA,USB3,0,46.5,FINESTEERING,2107,283093.750,02008000,471d,15824;INS_ALIGNMENT_COMPLETE,INS_RTKFIXED,37.37108790514,126.72336900394,8.2261,22.3000,0.0049,0.0045,0.0000,-0.407478337,-0.576861946,287.929394509,0.2139,0.1578,0.2812,0.0344,0.0343,0.0312,0.0796,0.0806,4.9028,0f000005,0*f255cd77\n\t", "INSPVAXA,USB3,0,49.5,FINESTEERING,2107,283094.250,02008000,471d,15824;INS_ALIGNMENT_COMPLETE,INS_RTKFIXED,37.37108790174,126.72336900960,8.2259,22.3000,0.0041,0.0045,-0.0005,-0.407655175,-0.578418030,287.928618080,0.2134,0.1577,0.2795,0.0344,0.0343,0.0312,0.0796,0.0805,4.9042,0f000005,0*67a4f1a6\n\t", "INSPVAXA,USB3,0,49.5,FINESTEERING,2107,283094.750,02008000,471d,15824;INS_ALIGNMENT_COMPLETE,INS_RTKFIXED,37.37108789686,126.72336901475,8.2257,22.3000,0.0044,0.0046,-0.0012,-0.406458944,-0.580608983,287.928943902,0.2134,0.1577,0.2795,0.0344,0.0343,0.0312,0.0796,0.0805,4.9042,0f000005,0*f975bb71\n\t", "DUALANTENNAHEADINGA,USB3,0,46.0,FINESTEERING,2107,283095.200,02008000,d426,15824;INSUFFICIENT_OBS,NONE,-1.000000000,0.000000000,0.000000000,0.0,0.000000000,0.000000000,\"631T\",15,2,2,2,04,00,20,00*3978f3e0\n\t", "INSPVAXA,USB3,0,46.0,FINESTEERING,2107,283095.750,02008000,471d,15824;INS_ALIGNMENT_COMPLETE,INS_RTKFIXED,37.37108789802,126.72336901889,8.2258,22.3000,0.0057,0.0037,-0.0015,-0.407856141,-0.581296268,287.930403916,0.2130,0.1576,0.2780,0.0344,0.0343,0.0312,0.0795,0.0805,4.9056,0f000005,0*89459e2d\n\t", "INSPVAXA,USB3,0,44.5,FINESTEERING,2107,283096.250,02000000,471d,15824;INS_ALIGNMENT_COMPLETE,INS_RTKFIXED,37.37108790052,126.72336901738,8.2259,22.3000,0.0066,0.0026,-0.0012,-0.409158540,-0.581176612,287.930571782,0.2126,0.1576,0.2766,0.0344,0.0343,0.0312,0.0795,0.0805,4.9071,0f000005,0*d38b9ae0\n\t", "INSPVAXA,USB3,0,44.5,FINESTEERING,2107,283096.750,02000000,471d,15824;INS_ALIGNMENT_COMPLETE,INS_RTKFIXED,37.37108790177,126.72336901650,8.2263,22.3000,0.0066,0.0025,-0.0011,-0.409708018,-0.580992332,287.931343125,0.2126,0.1576,0.2766,0.0344,0.0343,0.0312,0.0795,0.0805,4.9071,0f000005,0*11cd3564\n\t", "INSPVAXA,USB3,0,50.0,FINESTEERING,2107,283097.250,02000000,471d,15824;INS_ALIGNMENT_COMPLETE,INS_RTKFIXED,37.37108790174,126.72336901580,8.2265,22.3000,0.0063,0.0024,-0.0010,-0.411930313,-0.582541736,287.929452176,0.2123,0.1575,0.2753,0.0344,0.0343,0.0312,0.0795,0.0805,4.9086,0f000005,0*85d40b4e\n\t", "INSPVAXA,USB3,0,50.0,FINESTEERING,2107,283097.750,02000000,471d,15824;INS_ALIGNMENT_COMPLETE,INS_RTKFIXED,37.37108790027,126.72336901488,8.2267,22.3000,0.0062,0.0022,-0.0007,-0.412766504,-0.583030959,287.927282231,0.2123,0.1575,0.2753,0.0344,0.0343,0.0312,0.0795,0.0805,4.9086,0f000005,0*89dff8ff\n\t", "INSPVAXA,USB3,0,48.5,FINESTEERING,2107,283098.250,02000000,471d,15824;INS_ALIGNMENT_COMPLETE,INS_RTKFIXED,37.37108790003,126.72336901347,8.2268,22.3000,0.0066,0.0014,-0.0006,-0.413922974,-0.582701162,287.926560126,0.2120,0.1575,0.2742,0.0344,0.0343,0.0312,0.0795,0.0805,4.9101,0f000005,0*70ee257d\n\t", "INSPVAXA,USB3,0,48.5,FINESTEERING,2107,283098.750,02000000,471d,15824;INS_ALIGNMENT_COMPLETE,INS_RTKFIXED,37.37108789759,126.72336901204,8.2269,22.3000,0.0059,0.0011,-0.0001,-0.414260974,-0.583807411,287.925600594,0.2120,0.1575,0.2742,0.0344,0.0343,0.0312,0.0795,0.0805,4.9101,0f000005,0*03dc57a5\n\t", "INSPVAXA,USB3,0,49.0,FINESTEERING,2107,283099.250,02000000,471d,15824;INS_ALIGNMENT_COMPLETE,INS_RTKFIXED,37.37108789570,126.72336901200,8.2271,22.3000,0.0061,0.0012,0.0001,-0.415797201,-0.582658490,287.926983863,0.2118,0.1575,0.2731,0.0344,0.0343,0.0312,0.0795,0.0805,4.9116,0f000005,0*b658d869\n\t", "INSPVAXA,USB3,0,51.5,FINESTEERING,2107,283100.250,02000000,471d,15824;INS_ALIGNMENT_COMPLETE,INS_RTKFIXED,37.37108789328,126.72336901997,8.2271,22.3000,0.0052,0.0025,0.0001,-0.415319706,-0.581468435,287.925172452,0.2115,0.1574,0.2721,0.0344,0.0343,0.0312,0.0795,0.0805,4.9131,0f000005,0*eafa8938\n\t", "INSPVAXA,USB3,0,51.5,FINESTEERING,2107,283101.250,02000000,471d,15824;INS_ALIGNMENT_COMPLETE,INS_RTKFIXED,37.37108788280,126.72336902694,8.2267,22.3000,0.0032,0.0031,0.0001,-0.415895315,-0.578950026,287.923664941,0.2113,0.1574,0.2712,0.0344,0.0343,0.0312,0.0795,0.0805,4.9145,0f000005,0*44540dbc\n\t", "INSPVAXA,USB3,0,51.5,FINESTEERING,2107,283101.750,02000000,471d,15824;INS_ALIGNMENT_COMPLETE,INS_RTKFIXED,37.37108787688,126.72336902839,8.2270,22.3000,0.0029,0.0036,0.0002,-0.417826855,-0.580147759,287.923061019,0.2113,0.1574,0.2712,0.0344,0.0343,0.0312,0.0795,0.0805,4.9145,0f000005,0*aaec6ebb\n\t", "INSPVAXA,USB3,0,47.0,FINESTEERING,2107,283102.250,02000000,471d,15824;INS_ALIGNMENT_COMPLETE,INS_RTKFIXED,37.37108787301,126.72336903085,8.2270,22.3000,0.0026,0.0034,0.0000,-0.417491423,-0.580282079,287.923862604,0.2111,0.1574,0.2703,0.0344,0.0343,0.0312,0.0795,0.0805,4.9158,0f000005,0*ceb9045c\n\t", "INSPVAXA,USB3,0,47.0,FINESTEERING,2107,283102.750,02000000,471d,15824;INS_ALIGNMENT_COMPLETE,INS_RTKFIXED,37.37108787295,126.72336903129,8.2268,22.3000,0.0030,0.0034,0.0005,-0.416932840,-0.582279475,287.924574839,0.2111,0.1574,0.2703,0.0344,0.0343,0.0312,0.0795,0.0805,4.9158,0f000005,0*3c34a6bf\n\t", "INSPVAXA,USB3,0,48.5,FINESTEERING,2107,283103.750,02000000,471d,15824;INS_ALIGNMENT_COMPLETE,INS_RTKFIXED,37.37108788000,126.72336903510,8.2270,22.3000,0.0050,0.0045,0.0003,-0.414277574,-0.583463216,287.925982879,0.2110,0.1573,0.2695,0.0344,0.0343,0.0312,0.0795,0.0805,4.9172,0f000005,0*7ee9c1ee\n\t", "INSPVAXA,USB3,0,49.0,FINESTEERING,2107,283104.250,02000000,471d,15824;INS_ALIGNMENT_COMPLETE,INS_RTKFIXED,37.37108788419,126.72336903801,8.2270,22.3000,0.0052,0.0047,-0.0002,-0.414476277,-0.584193509,287.926239450,0.2108,0.1573,0.2688,0.0344,0.0343,0.0312,0.0795,0.0805,4.9186,0f000005,0*7089b505\n\t", "INSPVAXA,USB3,0,49.0,FINESTEERING,2107,283104.750,02000000,471d,15824;INS_ALIGNMENT_COMPLETE,INS_RTKFIXED,37.37108788145,126.72336903923,8.2266,22.3000,0.0045,0.0040,-0.0007,-0.415917885,-0.588202727,287.926434552,0.2108,0.1573,0.2688,0.0344,0.0343,0.0312,0.0795,0.0805,4.9186,0f000005,0*a8fd5de4\n\t", "INSPVAXA,USB3,0,48.0,FINESTEERING,2107,283105.250,02000000,471d,15824;INS_ALIGNMENT_COMPLETE,INS_RTKFIXED,37.37108788026,126.72336903795,8.2263,22.3000,0.0046,0.0032,-0.0010,-0.414361935,-0.591993164,287.925953212,0.2107,0.1573,0.2682,0.0344,0.0343,0.0312,0.0795,0.0805,4.9201,0f000005,0*118aea77\n\t", "INSPVAXA,USB3,0,48.0,FINESTEERING,2107,283105.750,02000000,471d,15824;INS_ALIGNMENT_COMPLETE,INS_RTKFIXED,37.37108788332,126.72336903309,8.2260,22.3000,0.0050,0.0029,-0.0017,-0.412327684,-0.591969420,287.923357283,0.2107,0.1573,0.2682,0.0344,0.0343,0.0312,0.0795,0.0805,4.9201,0f000005,0*6e4f183a\n\t", "INSPVAXA,USB3,0,48.5,FINESTEERING,2107,283106.250,02000000,471d,15824;INS_ALIGNMENT_COMPLETE,INS_RTKFIXED,37.37108788583,126.72336903030,8.2257,22.3000,0.0061,0.0025,-0.0021,-0.413322314,-0.593362730,287.923193741,0.2106,0.1573,0.2676,0.0344,0.0343,0.0312,0.0795,0.0805,4.9216,0f000005,0*8b1995f2\n\t", "INSPVAXA,USB3,0,48.5,FINESTEERING,2107,283106.750,02000000,471d,15824;INS_ALIGNMENT_COMPLETE,INS_RTKFIXED,37.37108788780,126.72336903040,8.2256,22.3000,0.0063,0.0024,-0.0014,-0.411919741,-0.593309816,287.922053260,0.2106,0.1573,0.2676,0.0344,0.0343,0.0312,0.0795,0.0805,4.9216,0f000005,0*86796b00\n\t", "INSPVAXA,USB3,0,49.0,FINESTEERING,2107,283108.250,02000000,471d,15824;INS_ALIGNMENT_COMPLETE,INS_RTKFIXED,37.37108788248,126.72336902361,8.2250,22.3000,0.0042,0.0015,-0.0018,-0.409863659,-0.598671820,287.918736221,0.2106,0.1573,0.2666,0.0344,0.0343,0.0312,0.0795,0.0805,4.9245,0f000005,0*9ed896c6\n\t", "INSPVAXA,USB3,0,49.0,FINESTEERING,2107,283108.750,02000000,471d,15824;INS_ALIGNMENT_COMPLETE,INS_RTKFIXED,37.37108788055,126.72336902250,8.2249,22.3000,0.0042,0.0020,-0.0022,-0.409039214,-0.598045025,287.918760673,0.2106,0.1573,0.2666,0.0344,0.0343,0.0312,0.0795,0.0805,4.9245,0f000005,0*7d4209e8\n\t", "INSPVAXA,USB3,0,49.0,FINESTEERING,2107,283109.250,02000000,471d,15824;INS_ALIGNMENT_COMPLETE,INS_RTKFIXED,37.37108788018,126.72336902226,8.2247,22.3000,0.0041,0.0020,-0.0021,-0.409961189,-0.600264889,287.916717631,0.2105,0.1573,0.2661,0.0344,0.0343,0.0312,0.0795,0.0805,4.9260,0f000005,0*bcf00a2d\n\t", "INSPVAXA,USB3,0,49.0,FINESTEERING,2107,283109.750,02000000,471d,15824;INS_ALIGNMENT_COMPLETE,INS_RTKFIXED,37.37108788128,126.72336902017,8.2243,22.3000,0.0038,0.0017,-0.0025,-0.411876741,-0.602713375,287.916096171,0.2105,0.1573,0.2661,0.0344,0.0343,0.0312,0.0795,0.0805,4.9260,0f000005,0*0e51d129\n\t", "INSPVAXA,USB3,0,47.0,FINESTEERING,2107,283110.250,02000000,471d,15824;INS_ALIGNMENT_COMPLETE,INS_RTKFIXED,37.37108788100,126.72336901819,8.2239,22.3000,0.0037,0.0018,-0.0030,-0.411621660,-0.604000034,287.914564647,0.2104,0.1573,0.2657,0.0344,0.0343,0.0312,0.0795,0.0805,4.9275,0f000005,0*d6cead36\n\t", "INSPVAXA,USB3,0,47.0,FINESTEERING,2107,283110.750,02000000,471d,15824;INS_ALIGNMENT_COMPLETE,INS_RTKFIXED,37.37108787882,126.72336901490,
